vi "ALTS-2015 UUT clamped.vi"(8 "error in":errorcluster, 11 "Station Cluster":T1) -> (0 "error out":errorcluster)   [LabVIEW 2013]
doc: "Copyright © 2005, Soliton Technologies.\nAll rights reserved."
uses:
  Controls/ALTS-2015 Station Cluster.ctl
  Controls/ALTS-2015 LV2GBL Station Info Options.ctl
  Controls/ALTS-2015 LV2GBL WorkOrder&SN Info Options.ctl
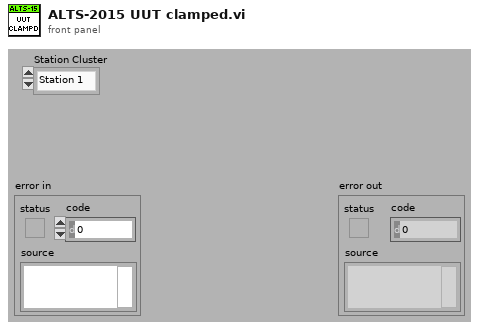
[diagram p1: front panel]
types:
  T1 = typedef "ALTS-2015 Station Cluster.ctl" = enum16{"Station 1", "Station 2", "Station 3", "Station 4"}
  T2 = typedef "ALTS-2015 LV2GBL Station Info Options.ctl" = enum16{"Init", "Read", "Read All", "Write Sensor ID", "Write  Work Order", "Write Serial Number", "Write Test Data", "Write Station Status", "Write Station Occupancy", "Write Station Test Type", "Write Rerun", "Write Load Decision", "Write Robot Action", "Clear All", "Clear Test Result"}
  T3 = typedef "ALTS-2015 LV2GBL WorkOrder&SN Info Options.ctl" = enum16{"Init", "Read all", "Write Work Order"}
  T4 = typedef "ALTS-2015 WorkOrder&SN Cluster.ctl" = cluster{"Work Order Number":string}
  T5 = typedef "ALTS-2015 Station Details.ctl" = cluster{"Station Number":string, "Work Order Number":string, "Sensor Name":string, "Pressure (PSI)":string, "Flow (SCCM)":string, "Test Time ":string, "Test Result":string, "Serial Number":string, "Station Status":T6, "SW assigned UUT":bool, "Rerun Count":i32, "Test Type":i32, "Load Decision":i32, "Robot Action":T7}
  T6 = typedef "ALTS-2015 Status Ring Indicator.ctl" = u16
  T7 = typedef "ALTS-2015 Robot Actions.ctl" = enum16{"Loading...", "Unloading...", "Reruning...", "No Action"}
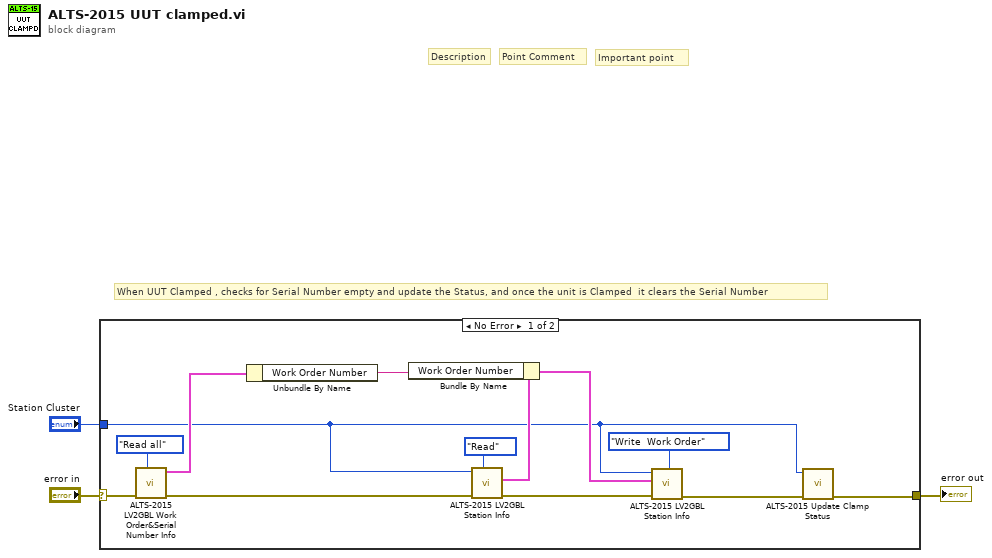
[diagram p0: block diagram]
diagram:
  # "When UUT Clamped , checks for Serial Number empty and update the Status, and once the unit is Clamped  it clears the Serial Number"
  # "Point Comment"
  # "Important point"
  # "Description"
  n1 = case shown="No Error" "error in" {
    selector: "error in" -> [w11 w17]
    tunnel: [w6 w17] -> w2
    tunnel: "Station Cluster" -> [w4 _]
    frame No Error {
      n2 = call "ALTS-2015 LV2GBL Work Order&Serial Number Info.vi"("Options"=ALTS-2015_LV2GBL_WorkOrder&SN_Info_Options."Read all", "error in"=w11) -> ("error out"=w8:errorcluster, "Work Order&SN Cluster Out"=w15:T4)  [unwired: 8 in]
      n3 = Unbundle By Name(w15) -> ("Work Order Number"=w9:string)
      n4 = call "ALTS-2015 LV2GBL Station Info.vi"("Options"=ALTS-2015_LV2GBL_Station_Info_Options."Read", "error in"=w8, "Station Cluster"=w4) -> ("error out"=w13:errorcluster, "Station Details"=w12:T5)  [unwired: 6 in, 1 out]
      n5 = Bundle By Name(cluster=w12, "Work Order Number"=w9) -> (w5:T5)
      n6 = call "ALTS-2015 LV2GBL Station Info.vi"("Options"=ALTS-2015_LV2GBL_Station_Info_Options."Write  Work Order", "error in"=w13, "Station"=w5, "Station Cluster"=w4) -> ("error out"=w7:errorcluster)  [unwired: 5 in, 2 out]
      n7 = call "ALTS-2015 Update Clamp Status.vi"("error in"=w7, "Station Cluster"=w4) -> ("error out"=w6:errorcluster)  [unwired: 9 in]
    }
    frame Error {
    }
  }
  "error out" <- w2
